vi "ANN Config.vi"() -> (0 "error out":errorcluster, 1 "error out 2":errorcluster, 2 "FPGA VI Reference Out 2":refnum<k20>, 3 "Refnum out":refnum<k20>, 4 "error out":errorcluster, 5 "Intial Bias\n& Weights":dbl[](array[numeric]))   [LabVIEW 2020]
uses:
  <vilib>/FPGAPlugInAG/IC-3173/niLvFpga_Open_IC-3173.vi
  <vilib>/rvi/interface/common/dynamic/niFpgaDynamicAddResources.vi
  <vilib>/FPGAPlugInAG/Dynamic/niLvFpga_Run_Dynamic.vi
  <vilib>/Utility/error.llb/Error Cluster From Error Code.vi
  <vilib>/rvi/errors/niLvFpgaAdjustHostInterfaceError.vi
  <vilib>/rvi/interface/nirviOpenFPGA/nirviOpenFPGA.xnode
  Recog-system - Copy (4)/FPGA Bitfiles/recog_FPGATarget_mainFPGAAnton_KcpJw9hx1Wg.lvbitx
  Recog-system - Copy (4)/ANN/mainFPGA_Anton.vi
  <vilib>/rvi/interface/nirviMethod/nirviMethod.xnode
  <vilib>/FPGAPlugInAG/Dynamic/niLvFpga_WriteFifo_Dynamic.vi
  <vilib>/rvi/errors/niLvFpgaMergeErrorWithErrorCode.vi
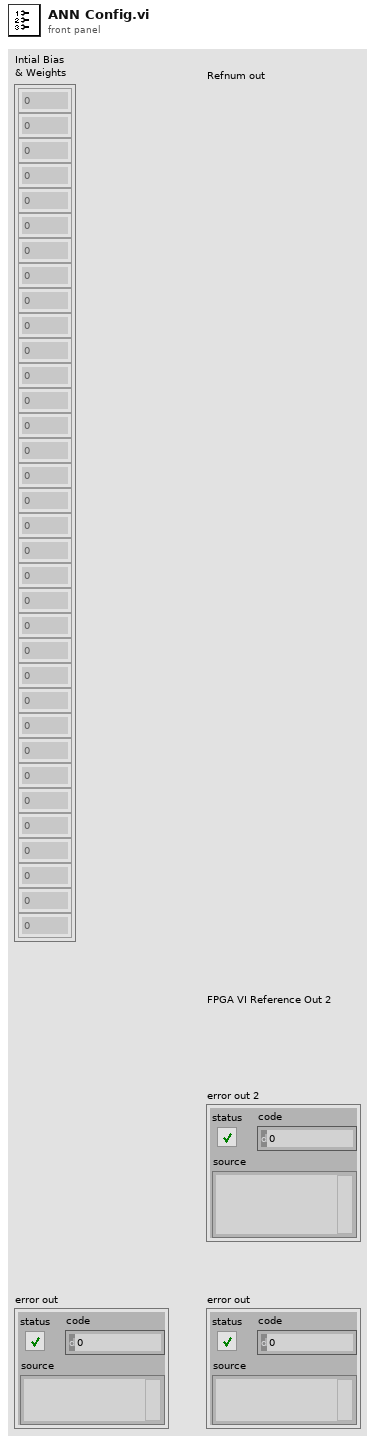
[diagram p1: front panel]
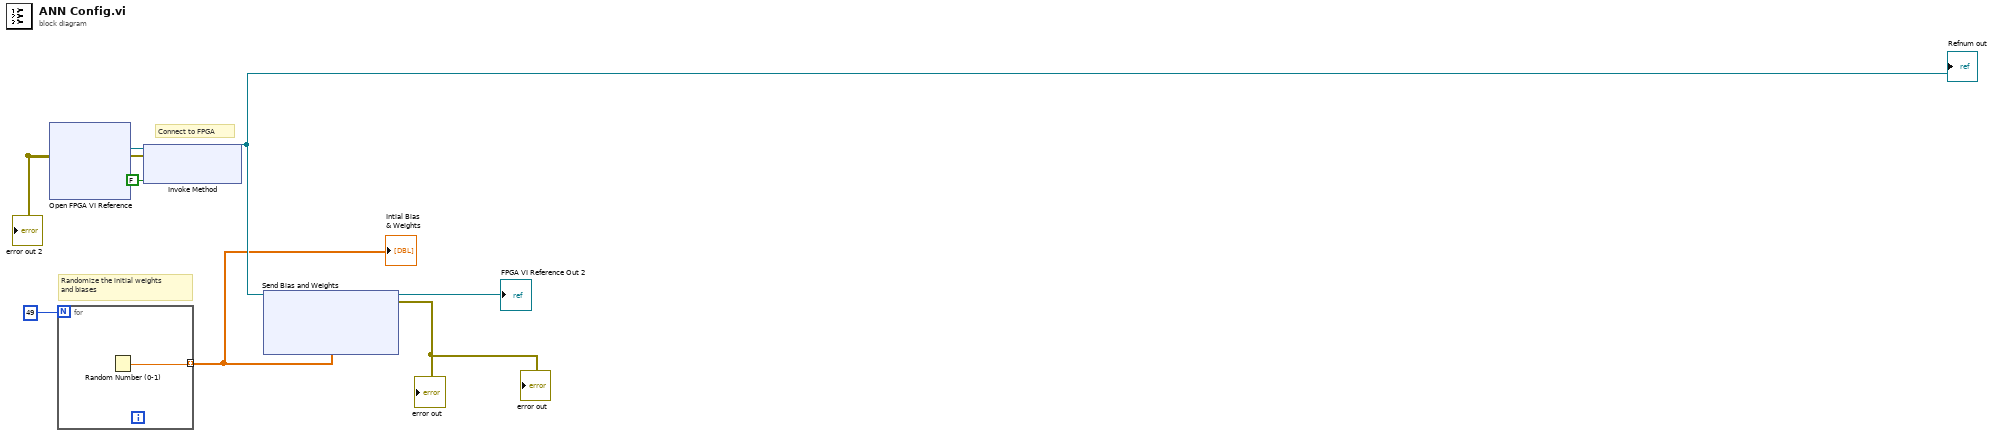
[diagram p0: block diagram]
diagram:
  # "Randomize the initial weights \nand biases"
  # "Connect to FPGA"
  n1 = xnode "Open FPGA VI Reference"() -> ("FPGA VI Reference Out"=w7:refnum<k20>, "error out"=w8:errorcluster)  [unwired: 2 in]
  "error out 2" <- w8
  n2 = for {
    N: 49 -> [_]
    tunnel: [w9] -> w1 mode=indexing
    n3 = Random Number (0-1)() -> (number: 0 to 1=w9:dbl)
  }
  "Intial Bias\n& Weights" <- w1
  n4 = xnode "Invoke Method"("FPGA VI Reference In"=w7, "error in"=w8, "Wait Until Done (F)"=FALSE) -> ("FPGA VI Reference Out"=w5:refnum<k20>)  [unwired: 1 out]
  "Refnum out" <- w5
  n5 = xnode "Send Bias and Weights"("FPGA VI Reference In"=w5, "Data"=w1) -> ("FPGA VI Reference Out"=→"FPGA VI Reference Out 2":refnum<k20>, "error out"=→"error out" →"error out":errorcluster)  [unwired: 2 in, 1 out]
